vi "SurreyBALDAS_Remote.vi"() -> ()   [LabVIEW 2022 SP3]
panel:
  in  "Quit":bool
  in  "Data Net Button":bool
  in  "data ABS button":bool
  in  "SigConSetup":bool
  in  "Numeric Zero(All Axis) button":bool caption="Numeric Zero(All Axis)"
  out "Roll gauge":dbl(slide) caption="100%             0                -100%" scale=-100.0..100.0
  out "Roll":dbl caption="N.m" format="%#.2f"
  out "Yaw gauge":dbl(slide) caption="100%             0                -100%" scale=-100.0..100.0
  out "Yaw":dbl caption="N.m" format="%#.2f"
  out "Side-force gauge":dbl(slide) caption="100%             0                -100%" scale=-100.0..100.0
  out "Side-Force":dbl caption="N" format="%#.2f"
  out "Drag Gauge":dbl(slide) caption="100%             0                -100%" scale=-100.0..100.0
  out "Drag":dbl caption="N" format="%#.2f"
  out "Pitch gauge":dbl(slide) caption="100%             0                -100%" scale=-100.0..100.0
  out "Pitch":dbl caption="N.m" format="%#.2f"
  out "Lift gauge":dbl(slide) caption="100%             0                -100%" scale=-100.0..100.0
  out "Lift":dbl caption="N" format="%#.2f"
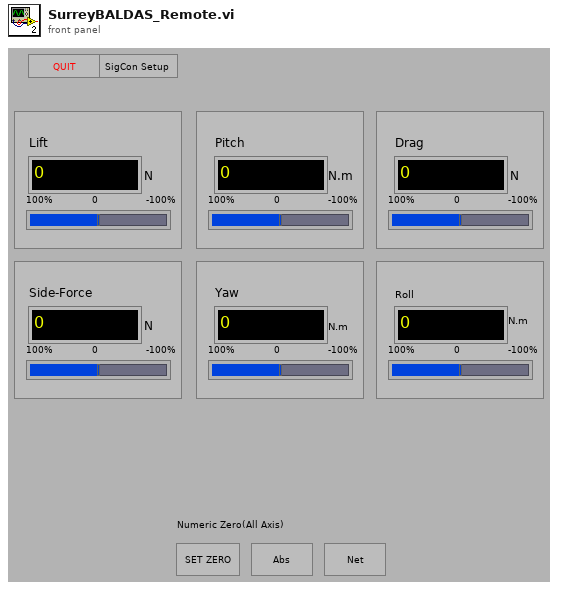
[diagram p1: front panel]
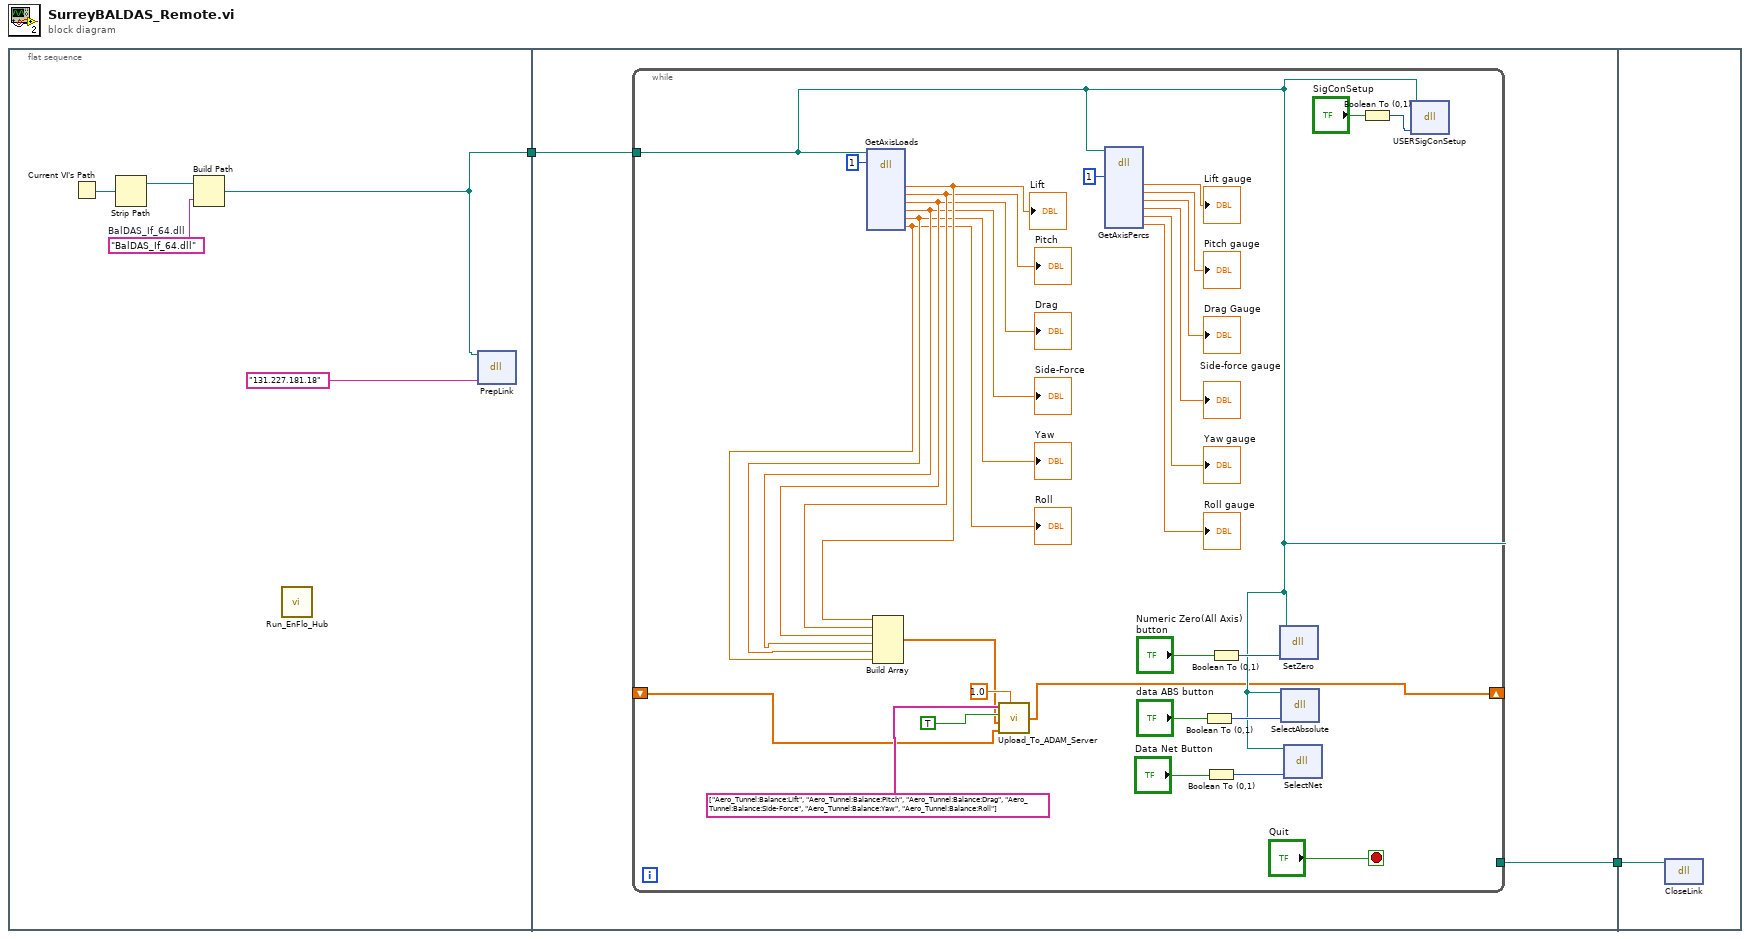
[diagram p0: block diagram]
diagram:
  n1 = flat-sequence {
    tunnel: [w3] -> w2
    tunnel: w2 -> [w9]
    tunnel: [w8] -> w1
    tunnel: w1 -> [w40]
    frame #0 {
      w4 = "BalDAS_If_64.dll"  # BalDAS_If_64.dll
      n2 = Current VI's Path() -> (path=w6:path)
      n3 = Strip Path(path=w6) -> (stripped path=w5:path)  [unwired: 1 out]
      n4 = Build Path(base path=w5, name or relative path=w4) -> (appended path=w3:path)
      n5 = call "Run_EnFlo_Hub.vi"() -> ()  [unwired: 7 in, 1 out]
      n6 = dll-call lib="C:/Aerotech/SurreyBaldas/BalDAS_If.dl" fn="PrepLink"(path in=w3, "IPAddress"="131.227.181.18") -> ()  [unwired: 2 in, 4 out]
    }
    frame #1 {
      n7 = while {
        tunnel: w9 -> [w22]
        tunnel: [w22] -> w8
        shift-right: [w10] -> _
        shift-left: _ -> [w11]
        stop <- "Quit" stop-if-true
        n8 = dll-call lib="C:/Aerotech/SurreyBaldas/BalDAS_If.dl" fn="GetAxisLoads"(path in=w22, "Enable"=1) -> ("Lift"=w21:dbl, "Pitch"=w20:dbl, "Drag"=w19:dbl, "side"=w18:dbl, "Yaw"=w17:dbl, "Roll"=w16:dbl)  [unwired: 3 in, 9 out]
        "Lift" <- w21
        "Pitch" <- w20
        "Drag" <- w19
        "Side-Force" <- w18
        "Yaw" <- w17
        "Roll" <- w16
        n9 = Build Array(w21, w20, w19, w18, w17, w16) -> (w12:dbl[])
        n10 = call "Upload_To_ADAM_Server.vi"("Averaging Period (s)"=1.0, "Shift In"=w11, "Channel Values"=w12, "Give Variance"=TRUE, "Channel Names"=string[] ["Aero_Tunnel:Balance:Lift", "Aero_Tunnel:Balance:Pitch", "Aero_Tunnel:Balance:Drag", "Aero_Tunnel:Balance:Side-Force", "Aero_Tunnel:Balance:Yaw", "Aero_Tunnel:Balance:Roll"]) -> ("Shift Out"=w10:dbl[])  [unwired: 1 in]
        n11 = dll-call lib="C:/Aerotech/SurreyBaldas/BalDAS_If.dl" fn="GetAxisPercs"(path in=w22, "Enable"=1) -> ("Lift"=→"Lift gauge":dbl, "Pitch"=→"Pitch gauge":dbl, "Drag"=→"Drag Gauge":dbl, "side"=→"Side-force gauge":dbl, "Yaw"=→"Yaw gauge":dbl, "Roll"=→"Roll gauge":dbl)  [unwired: 3 in, 9 out]
        n12 = Boolean To (0,1)(Boolean="data ABS button") -> (0, 1=w25:i16)
        n13 = Boolean To (0,1)(Boolean="Data Net Button") -> (0, 1=w28:i16)
        n14 = Boolean To (0,1)(Boolean="Numeric Zero(All Axis) button") -> (0, 1=w31:i16)
        n15 = dll-call lib="C:/Aerotech/SurreyBaldas/BalDAS_If.dl" fn="SetZero"(path in=w22, "Enable"=w31) -> ()  [unwired: 2 in, 4 out]
        n16 = dll-call lib="C:/Aerotech/SurreyBaldas/BalDAS_If.dl" fn="SelectAbsolute"(path in=w22, "Enable"=w25) -> ()  [unwired: 2 in, 4 out]
        n17 = dll-call lib="C:/Aerotech/SurreyBaldas/BalDAS_If.dl" fn="SelectNet"(path in=w22, "Enable"=w28) -> ()  [unwired: 2 in, 4 out]
        n18 = Boolean To (0,1)(Boolean="SigConSetup") -> (0, 1=w23:i16)
        n19 = dll-call lib="C:/Aerotech/SurreyBaldas/BalDAS_If.dl" fn="USERSigConSetup"(path in=w22, "Enable"=w23) -> ()  [unwired: 2 in, 4 out]
      }
    }
    frame #2 {
      n20 = dll-call lib="C:/Aerotech/SurreyBaldas/BalDAS_If.dl" fn="CloseLink"(path in=w40) -> ()  [unwired: 2 in, 3 out]
    }
  }
